vi "combine1dArrays.vi"(10 "Array 2":variant[](array[variant]), 11 "Array 1":variant[](array[variant])) -> (3 "Combined Array Out":variant[](array[variant]))   [LabVIEW 2013]
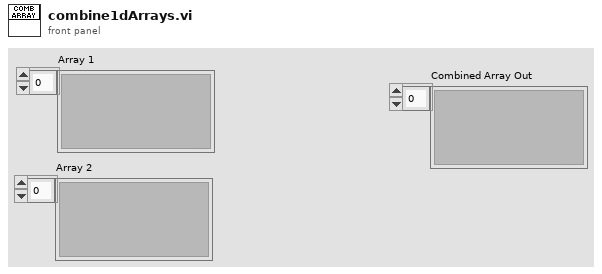
[diagram p1: front panel]
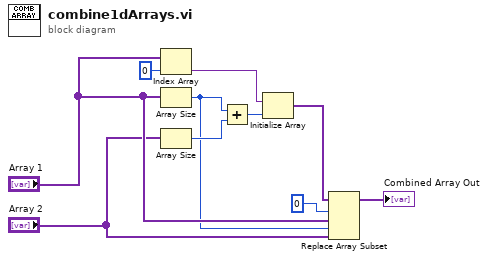
[diagram p0: block diagram]
diagram:
  n1 = Index Array(array="Array 1", index=0) -> (element=w2:variant)
  n2 = Array Size(array="Array 1") -> (size(s)=w4:i32)
  n3 = Array Size(array="Array 2") -> (size(s)=w10:i32)
  n4 = Add(x=w4, y=w10) -> (x+y=w9:i32)
  n5 = Initialize Array(w2, w9) -> (w7:variant[])
  n6 = Replace Array Subset(array=w7, new element #1="Array 1", index #1=0 ("index"), new element #2="Array 2", index #2=w4) -> (→"Combined Array Out":variant[])
